vi "test-Pose-Error.vi"() -> ()   [LabVIEW 2019]
uses:
  PathExecution_Library/POSE.ctl
  PathExecution_Library/TRANSLATION.ctl
  PathExecution_Library/ROTATION.ctl
  PathExecution_Library/Conv_AngleDegrees_Heading.vi
  PathExecution_Library/PathExecution_Library.lvlib
panel:
  out "Err Pose 2":T1
  out "Cur Pose 2":T1
  in  "LeftDist-Feet":dbl
  in  "RightDist-Feet":dbl
  in  "Reset":bool
  in  "Gyro-Deg":dbl
  out "Cur Pose":T1
  out "Des Pose":T1
  in  "Ang 2":dbl
  in  "Y 2":dbl
  in  "Cur X 2":dbl
  in  "Ang":dbl
  in  "Y":dbl
  in  "Des X":dbl
  in  "Next Step":bool
  out "Err Pose":T1
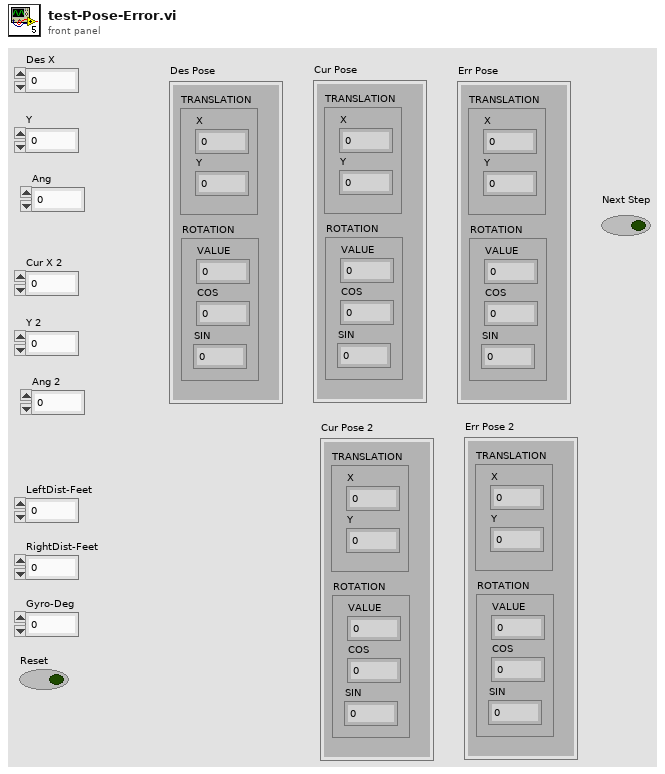
[diagram p1: front panel]
types:
  T1 = typedef "PathExecution_Library.lvlib/POSE.ctl" = cluster{"TRANSLATION":T2, "ROTATION":T3}
  T2 = typedef "PathExecution_Library.lvlib/TRANSLATION.ctl" = cluster{"X":dbl, "Y":dbl}
  T3 = typedef "PathExecution_Library.lvlib/ROTATION.ctl" = cluster{"VALUE":dbl, "COS":dbl, "SIN":dbl}
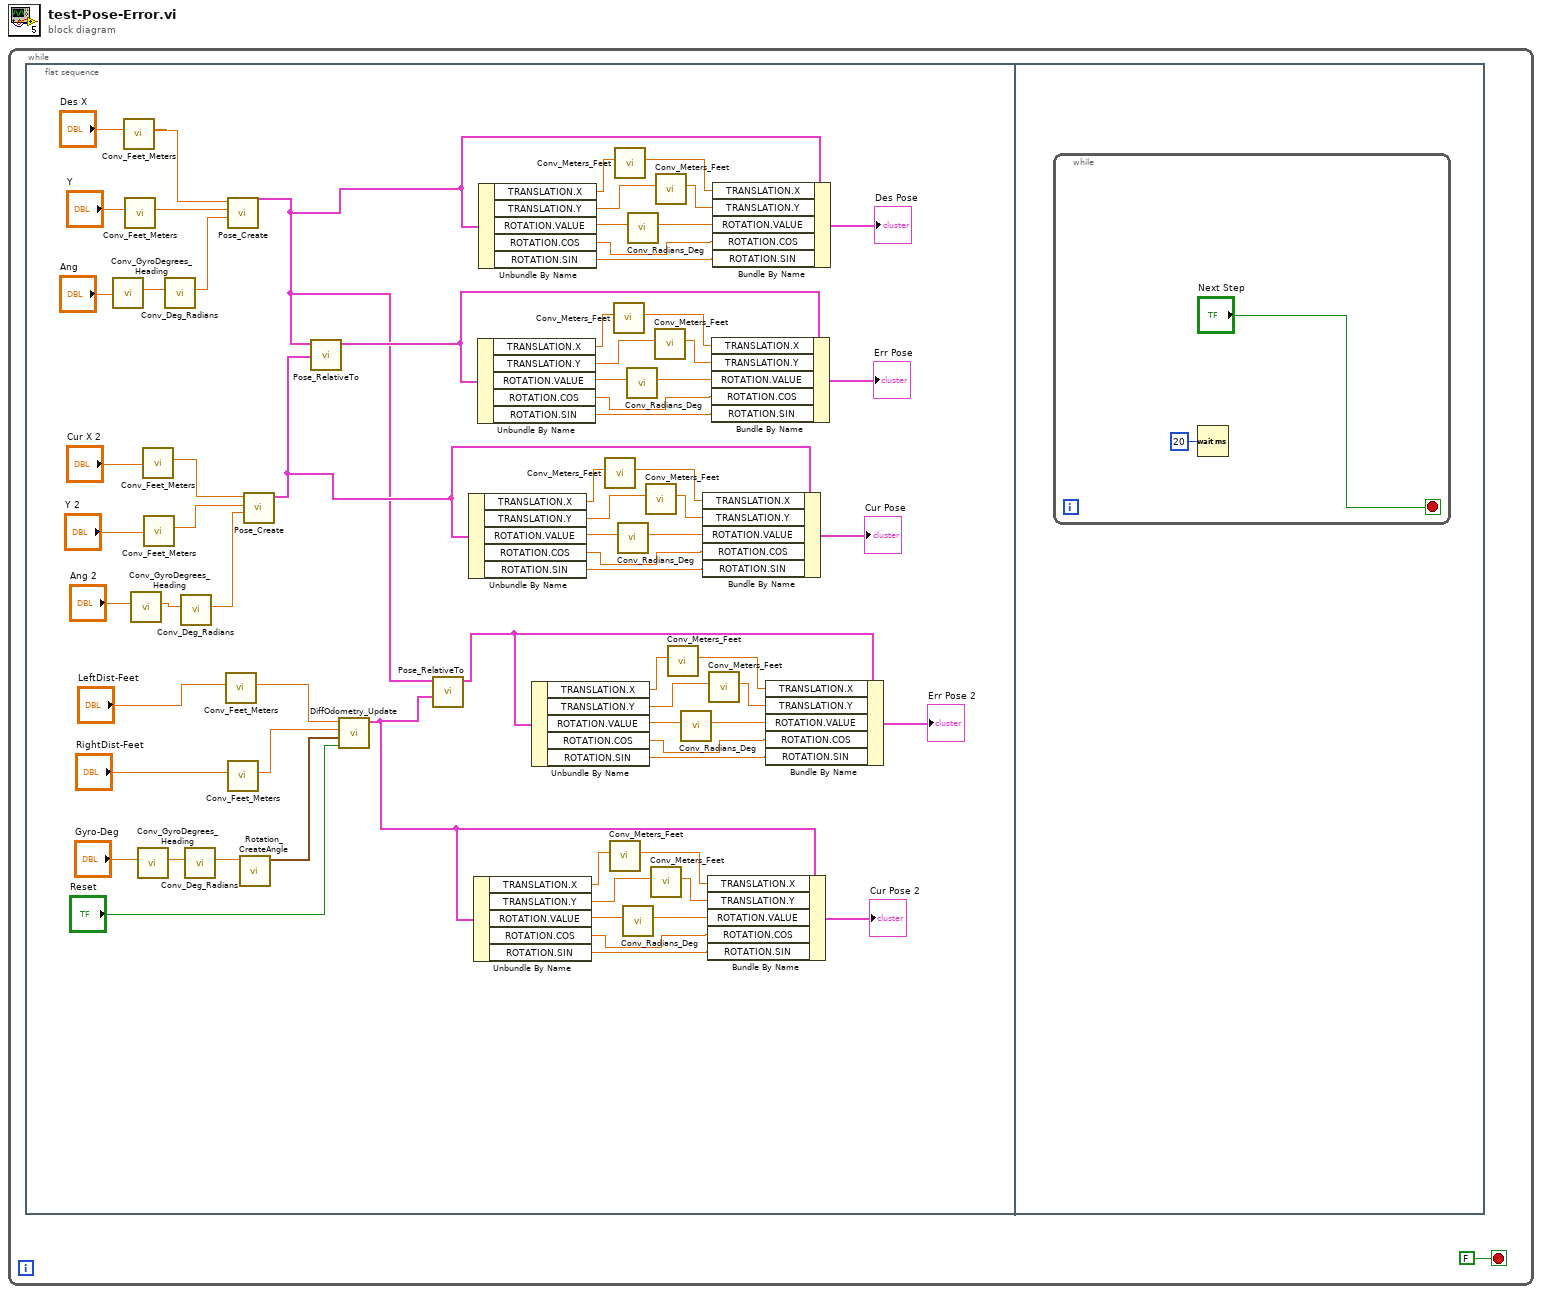
[diagram p0: block diagram]
diagram:
  n1 = while {
    stop <- FALSE stop-if-true
    n2 = flat-sequence {
      frame #0 {
        n3 = call "Conv_GyroDegrees_Heading.vi"("GyroDegrees"="Ang") -> ("HeadingDegrees"=w65:dbl)  [unwired: 10 in]
        n4 = call "Conv_Feet_Meters.vi"("Feet"="Des X") -> ("Meters"=w51:dbl)  [unwired: 10 in]
        n5 = call "Conv_Feet_Meters.vi"("Feet"="Y") -> ("Meters"=w60:dbl)  [unwired: 10 in]
        n6 = call "Conv_GyroDegrees_Heading.vi"("GyroDegrees"="Ang 2") -> ("HeadingDegrees"=w64:dbl)  [unwired: 10 in]
        n7 = call "Conv_GyroDegrees_Heading.vi"("GyroDegrees"="Gyro-Deg") -> ("HeadingDegrees"=w25:dbl)  [unwired: 10 in]
        n8 = call "Conv_Feet_Meters.vi"("Feet"="Cur X 2") -> ("Meters"=w55:dbl)  [unwired: 10 in]
        n9 = call "Conv_Feet_Meters.vi"("Feet"="Y 2") -> ("Meters"=w54:dbl)  [unwired: 10 in]
        n10 = call "Conv_Deg_Radians.vi"("Degress"=w65) -> ("Radians"=w59:dbl)  [unwired: 10 in]
        n11 = call "Conv_Deg_Radians.vi"("Degress"=w64) -> ("Radians"=w53:dbl)  [unwired: 10 in]
        n12 = call "Conv_Deg_Radians.vi"("Degress"=w25) -> ("Radians"=w24:dbl)  [unwired: 10 in]
        n13 = call "Conv_Feet_Meters.vi"("Feet"="LeftDist-Feet") -> ("Meters"=w30:dbl)  [unwired: 10 in]
        n14 = call "Pose_Create.vi"("Heading"=w59, "Y"=w60, "X"=w51) -> ("out POSe"=w12:T1)  [unwired: 8 in]
        n15 = call "Conv_Feet_Meters.vi"("Feet"="RightDist-Feet") -> ("Meters"=w31:dbl)  [unwired: 10 in]
        n16 = call "Rotation_CreateAngle.vi"("Angle"=w24) -> ("ROTATION"=w26:T3)  [unwired: 10 in]
        n17 = call "Pose_Create.vi"("Heading"=w53, "Y"=w54, "X"=w55) -> ("out POSe"=w32:T1)  [unwired: 8 in]
        n18 = call "Pose_RelativeTo.vi"("other POSE"=w32, "in POSE"=w12) -> ("out POSE"=w52:T1)  [unwired: 9 in]
        n19 = call "DiffOdometry_Update.vi"("Reset"="Reset", "Heading"=w26, "RightDistance"=w31, "LeftDistance"=w30) -> ("CurrentRelativePose"=w13:T1)  [unwired: 7 in]
        n20 = call "Pose_RelativeTo.vi"("other POSE"=w13, "in POSE"=w12) -> ("out POSE"=w2:T1)  [unwired: 9 in]
        n21 = Unbundle By Name(w32) -> ("TRANSLATION.X"=w40:dbl, "TRANSLATION.Y"=w39:dbl, "ROTATION.VALUE"=w41:dbl, "ROTATION.COS"=w37:dbl, "ROTATION.SIN"=w36:dbl)
        n22 = Unbundle By Name(w13) -> ("TRANSLATION.X"=w22:dbl, "TRANSLATION.Y"=w21:dbl, "ROTATION.VALUE"=w23:dbl, "ROTATION.COS"=w19:dbl, "ROTATION.SIN"=w18:dbl)
        n23 = Unbundle By Name(w52) -> ("TRANSLATION.X"=w73:dbl, "TRANSLATION.Y"=w72:dbl, "ROTATION.VALUE"=w74:dbl, "ROTATION.COS"=w70:dbl, "ROTATION.SIN"=w69:dbl)
        n24 = Unbundle By Name(w12) -> ("TRANSLATION.X"=w49:dbl, "TRANSLATION.Y"=w48:dbl, "ROTATION.VALUE"=w50:dbl, "ROTATION.COS"=w46:dbl, "ROTATION.SIN"=w45:dbl)
        n25 = Unbundle By Name(w2) -> ("TRANSLATION.X"=w10:dbl, "TRANSLATION.Y"=w9:dbl, "ROTATION.VALUE"=w11:dbl, "ROTATION.COS"=w7:dbl, "ROTATION.SIN"=w6:dbl)
        n26 = call "Conv_Meters_Feet.vi"("Meters"=w40) -> ("Feet"=w34:dbl)  [unwired: 10 in]
        n27 = call "Conv_Meters_Feet.vi"("Meters"=w22) -> ("Feet"=w16:dbl)  [unwired: 10 in]
        n28 = call "Conv_Meters_Feet.vi"("Meters"=w73) -> ("Feet"=w67:dbl)  [unwired: 10 in]
        n29 = call "Conv_Meters_Feet.vi"("Meters"=w49) -> ("Feet"=w43:dbl)  [unwired: 10 in]
        n30 = call "Conv_Radians_Deg.vi"("Radians"=w41) -> ("Degrees"=w38:dbl)  [unwired: 10 in]
        n31 = call "Conv_Radians_Deg.vi"("Radians"=w23) -> ("Degrees"=w20:dbl)  [unwired: 10 in]
        n32 = call "Conv_Radians_Deg.vi"("Radians"=w74) -> ("Degrees"=w71:dbl)  [unwired: 10 in]
        n33 = call "Conv_Radians_Deg.vi"("Radians"=w50) -> ("Degrees"=w47:dbl)  [unwired: 10 in]
        n34 = call "Conv_Meters_Feet.vi"("Meters"=w39) -> ("Feet"=w35:dbl)  [unwired: 10 in]
        n35 = call "Conv_Meters_Feet.vi"("Meters"=w21) -> ("Feet"=w17:dbl)  [unwired: 10 in]
        n36 = call "Conv_Meters_Feet.vi"("Meters"=w72) -> ("Feet"=w68:dbl)  [unwired: 10 in]
        n37 = call "Conv_Meters_Feet.vi"("Meters"=w48) -> ("Feet"=w44:dbl)  [unwired: 10 in]
        n38 = call "Conv_Meters_Feet.vi"("Meters"=w10) -> ("Feet"=w4:dbl)  [unwired: 10 in]
        n39 = call "Conv_Radians_Deg.vi"("Radians"=w11) -> ("Degrees"=w8:dbl)  [unwired: 10 in]
        n40 = Bundle By Name(cluster=w32, "TRANSLATION.X"=w34, "TRANSLATION.Y"=w35, "ROTATION.VALUE"=w38, "ROTATION.COS"=w37, "ROTATION.SIN"=w36) -> (→"Cur Pose":T1)
        n41 = Bundle By Name(cluster=w13, "TRANSLATION.X"=w16, "TRANSLATION.Y"=w17, "ROTATION.VALUE"=w20, "ROTATION.COS"=w19, "ROTATION.SIN"=w18) -> (→"Cur Pose 2":T1)
        n42 = call "Conv_Meters_Feet.vi"("Meters"=w9) -> ("Feet"=w5:dbl)  [unwired: 10 in]
        n43 = Bundle By Name(cluster=w52, "TRANSLATION.X"=w67, "TRANSLATION.Y"=w68, "ROTATION.VALUE"=w71, "ROTATION.COS"=w70, "ROTATION.SIN"=w69) -> (→"Err Pose":T1)
        n44 = Bundle By Name(cluster=w12, "TRANSLATION.X"=w43, "TRANSLATION.Y"=w44, "ROTATION.VALUE"=w47, "ROTATION.COS"=w46, "ROTATION.SIN"=w45) -> (→"Des Pose":T1)
        n45 = Bundle By Name(cluster=w2, "TRANSLATION.X"=w4, "TRANSLATION.Y"=w5, "ROTATION.VALUE"=w8, "ROTATION.COS"=w7, "ROTATION.SIN"=w6) -> (→"Err Pose 2":T1)
      }
      frame #1 {
        n46 = while {
          stop <- "Next Step" stop-if-true
          n47 = Wait (ms)(milliseconds to wait=u32 20) -> ()  [unwired: 1 out]
        }
      }
    }
  }
